vi "SEN_Loop.vi"() -> ()   [LabVIEW 2020, in "PigeonIMU_SEN_ts.lvlib"]
uses:
  PigeonIMU_SEN_ts.lvlib
  <vilib>/Rock Robotics/WPI/ThirdParty/Phoenix-LabVIEW/Pigeon2/controls/CTRE_Phoenix_Pigeon2_Configurables.ctl
  Cluster_CMD_SEN_Data.ctl
  Shared Code/TypeDefs/Cluster_Unity Yaw-Pitch-Roll.ctl
  Shared Code/TypeDefs/Dial_Compase heading unit circle CCW positive.ctl
  ENUM_SEN_State.ctl
  <vilib>/Rock Robotics/WPI/ThirdParty/Phoenix-LabVIEW/Pigeon IMU/CTRE_PigeonIMU_DeviceRef.ctl
  <vilib>/Rock Robotics/WPI/ThirdParty/Phoenix-LabVIEW/Pigeon IMU/CTRE_PigeonIMU_ConnectionType.ctl
  ENUM_SEN_Action.ctl
  ca1e8ace-5cb3-4d4b-8a00-bfa7a3df30b2.vi
  Global_CMD_SEN_Data In.vi
  RoboRIO Utilities/Global_STOP.vi
  Global_SEN_Data Out.vi
  <vilib>/Rock Robotics/WPI/ThirdParty/Phoenix-LabVIEW/Pigeon2/CTRE_Phoenix_Pigeon2_GetGravityVector.vi
  <vilib>/Rock Robotics/WPI/ThirdParty/Phoenix-LabVIEW/Pigeon IMU/CTRE_PigeonIMU_GetRawGyro.vi
  <vilib>/Rock Robotics/WPI/ThirdParty/Phoenix-LabVIEW/Pigeon IMU/CTRE_PigeonIMU_GetFusedHeading.vi
  <vilib>/Rock Robotics/WPI/ThirdParty/Phoenix-LabVIEW/Pigeon IMU/CTRE_PigeonIMU_GetBiasedAccelerometer.vi
panel:
  out "Pigeon Running":bool
  out "YawPitchRoll":T1 {"Roll" scale format="%.3f"; "Pitch" scale format="%.3f"; "Yaw" scale format="%.3f"}
  in  "CMD_SEN_Pigeon_Data":T3
  in  "Set Values":bool
  in  "Pigeon2 Config":T4
  out "Pigeon Ready":bool
  out "Pigeon Enabled":bool
  out "Cycle Time (S)":dbl format="%.3g"
  # "Yaw Angle needed to reach the current orientation in degrees"
  # "Configures the mounting pose of the Pigeon2\nThis is the yaw-pitch-roll teh Pigeon2 underwent to get to its current orientation,\n referenced from the robot's point of view\nThis is only necessary if the Pigeon2 is mounted at an exotic angle near the gimbal lock point or not forward.\nIf the pigeon is relatively flat and pointed forward, this is not needed"
  # "Pitch Angle needed to reach the current orientation in degrees"
  # "Roll Angle needed to reach the current orientation in degrees"
  # "Disables the temperature compensation\nfrom the Pigeon2. It is recommended that\nthis remains false"
  # "Disables the no-motion calibration from the\nPigeon2. It is recommended that this \nremains false"
  # "Enables the compass for Pigeon2\nThis is not recommended for any indoor robotics"
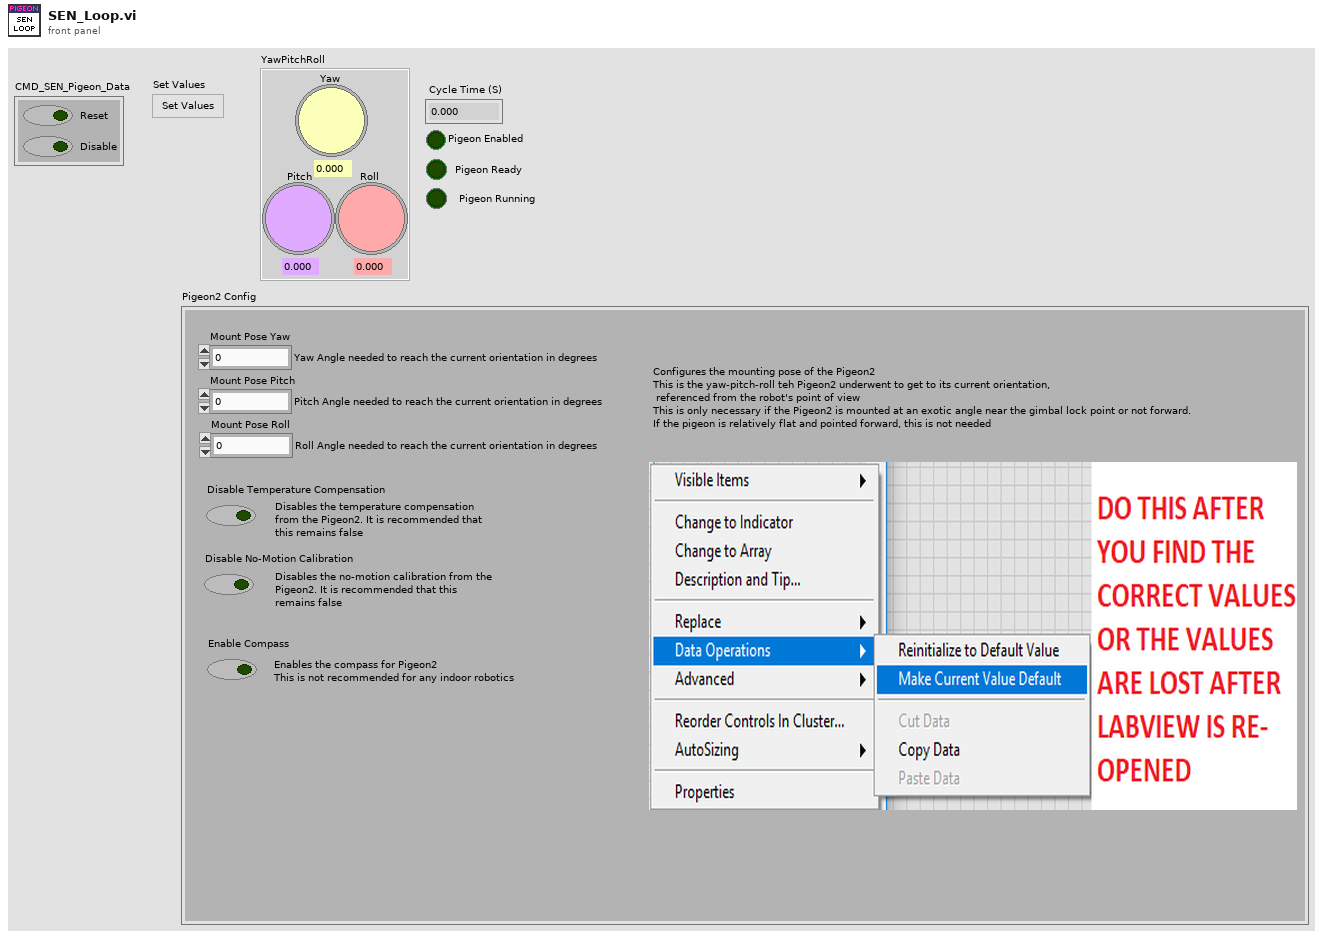
[diagram p1: front panel]
types:
  T1 = typedef "Cluster_Unity Yaw-Pitch-Roll.ctl" = cluster{"Yaw":T2, "Pitch":T2, "Roll":T2}
  T2 = typedef "Dial_Compase heading unit circle CCW positive.ctl" = dbl
  T3 = typedef "PigeonIMU_SEN_ts.lvlib/Cluster_CMD_SEN_Data.ctl" = cluster{"Reset":bool, "Disable":bool}
  T4 = typedef "CTRE_Phoenix_Pigeon2_Configurables.ctl" = cluster{"Mount Pose Yaw":dbl, "Mount Pose Pitch":dbl, "Mount Pose Roll":dbl, "Disable Temperature Compensation":bool, "Disable No-Motion Calibration":bool, "Enable Compass":bool}
  T5 = cluster{"Heading":dbl, "Valid?":bool, "Fusing?":bool}
  T6 = typedef "CTRE_PigeonIMU_DeviceRef.ctl" = cluster{"DeviceStatus":errorcluster, "Device Number":u8, "Type":T7, "Device ID":u32, "Handle":u64, "UsageFrame":u32, "Library Path":path}
  T7 = typedef "CTRE_PigeonIMU_ConnectionType.ctl" = u32
  T8 = typedef "PigeonIMU_SEN_ts.lvlib/ENUM_SEN_State.ctl" = enum16{"Starting", "Reseting", "Enableing", "Disabeling", "Shutting Down"}
  T9 = cluster{"PigeonIMUDevRef":T6, "State":T8, "Previous State":T8, "Current Time":timestamp, "Previous Time":timestamp, "Start Time":timestamp, "Target Time (ms)":u32, "Cycle Time(S)":dbl, "Reset":bool, "Yaw Pitch Roll":T1, "Fused Heading":cluster{"Heading":dbl, "Valid?":bool, "Fusing?":bool}, "IMU Ready":bool, "Swing Threshold":dbl, "Swinging":bool, "Swing Array Size":i32, "CMD_SEN_Pigeon_Data":T3}
  T10 = typedef "PigeonIMU_SEN_ts.lvlib/ENUM_SEN_Action.ctl" = enum16{"No Action", "Reset Time", "Zero Heading", "Read Heading", "Read Raw ", "Configure IMU", "Check IMU Reset", "Set Enable Cycle Time", "Set Disable Cycle Time"}
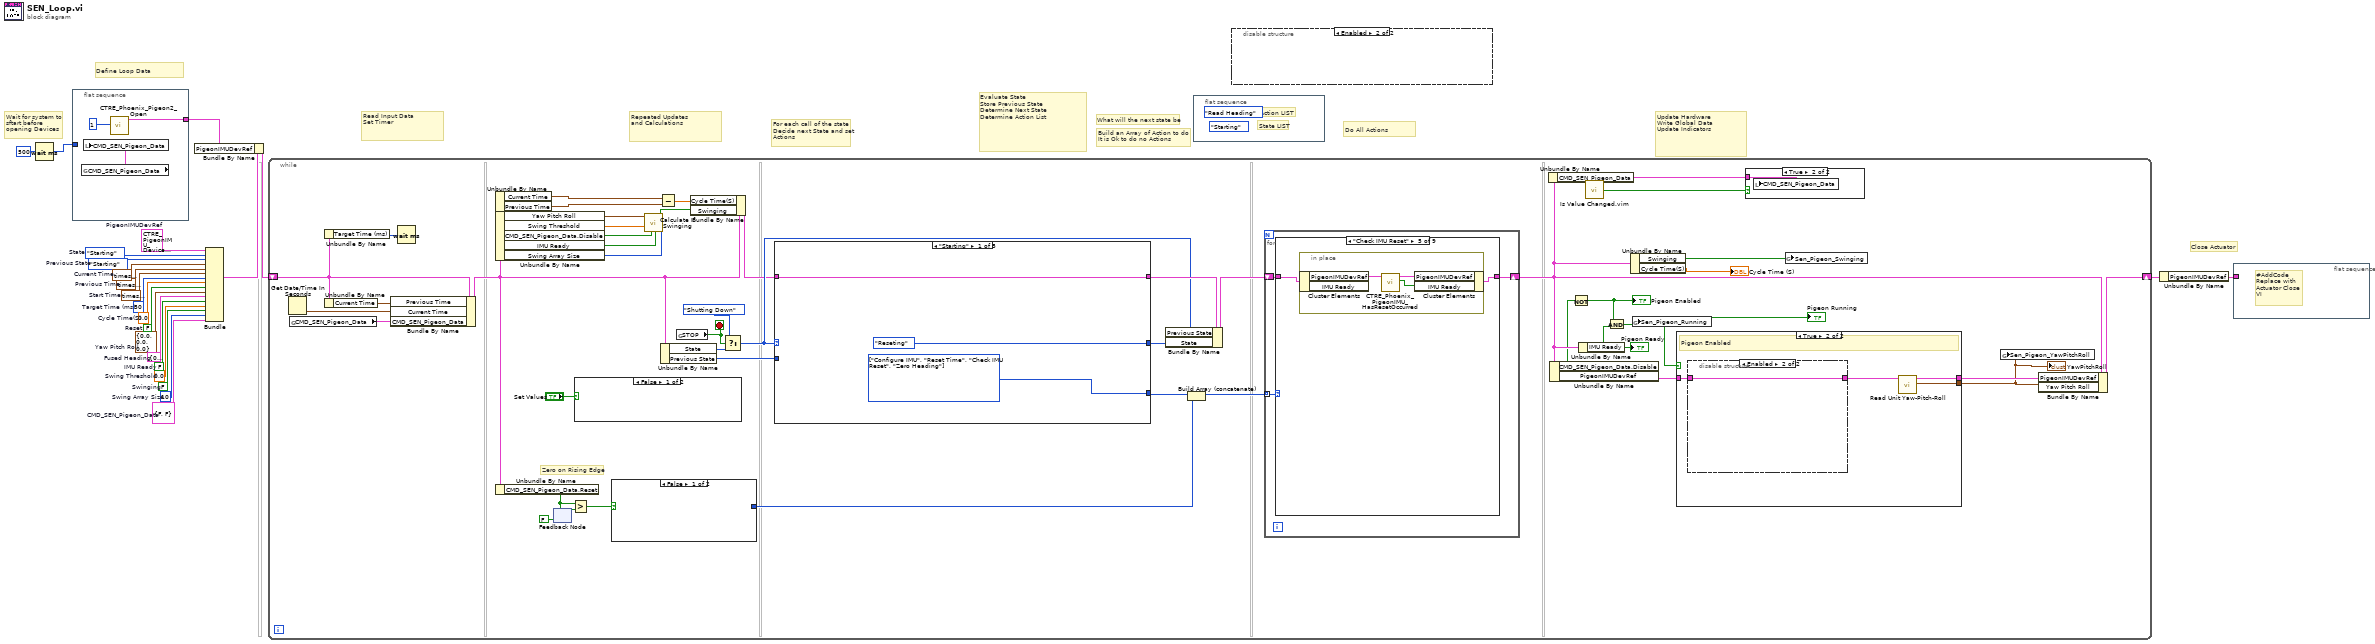
[diagram p0: block diagram]
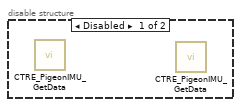
[diagram p2: hidden frame]
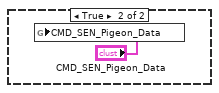
[diagram p4: hidden frame]
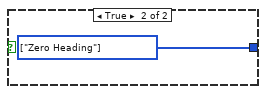
[diagram p5: hidden frame]
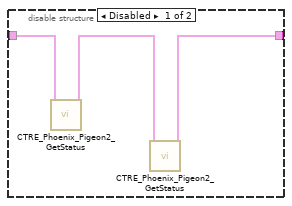
[diagram p7: hidden frame]
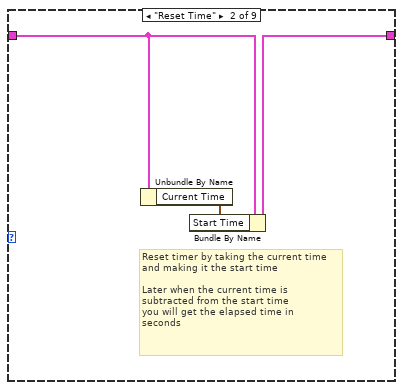
[diagram p9: hidden frame]
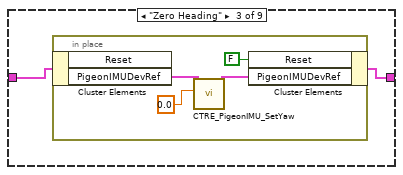
[diagram p10: hidden frame]
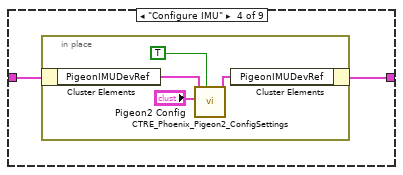
[diagram p11: hidden frame]
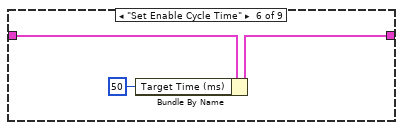
[diagram p12: hidden frame]
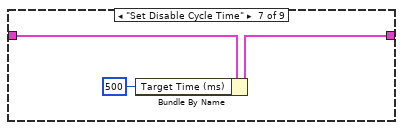
[diagram p13: hidden frame]
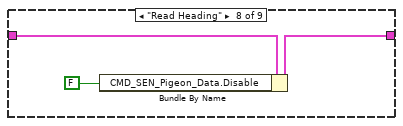
[diagram p14: hidden frame]
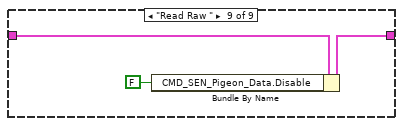
[diagram p15: hidden frame]
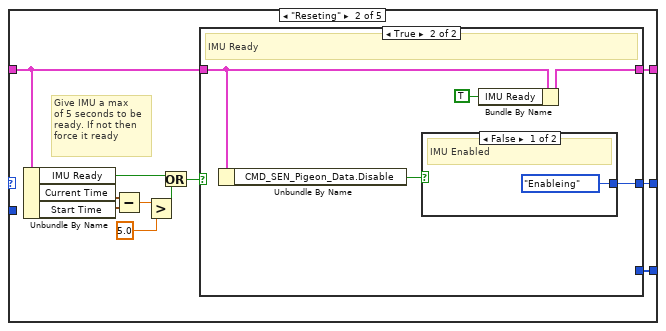
[diagram p16: hidden frame]
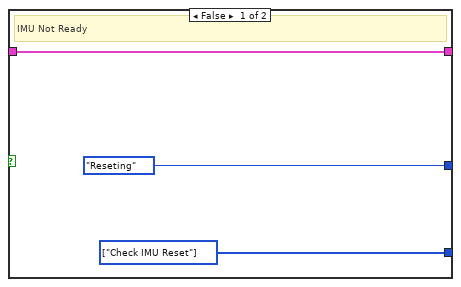
[diagram p17: hidden frame]
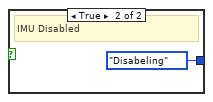
[diagram p18: hidden frame]
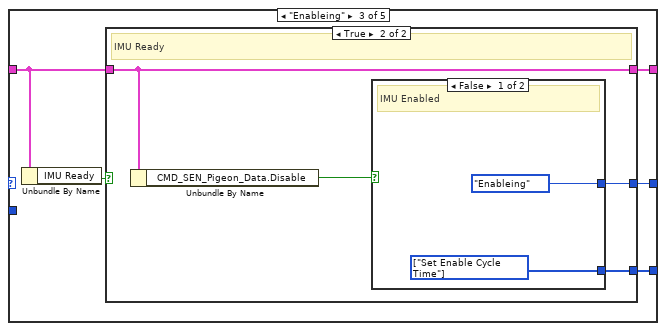
[diagram p19: hidden frame]
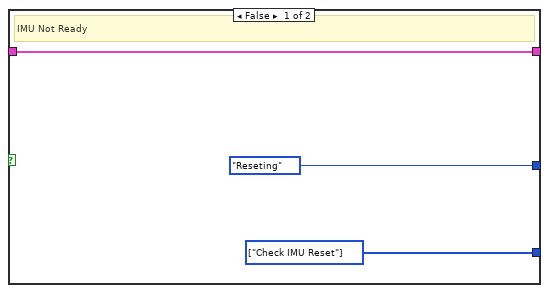
[diagram p20: hidden frame]
diagram:
  w1 = T1 {"Yaw"=0.0, "Pitch"=0.0, "Roll"=0.0}  # Yaw Pitch Roll
  w2 = T3 {"Reset"=FALSE, "Disable"=FALSE}  # CMD_SEN_Pigeon_Data
  w3 = 10  # Swing Array Size
  w4 = FALSE  # Swinging
  w5 = 0.0  # Swing Threshold
  w6 = FALSE  # IMU Ready
  w7 = T5 {"Heading"=0.0, "Valid?"=FALSE, "Fusing?"=FALSE}  # Fused Heading
  w8 = T6 {"DeviceStatus"={"status"=FALSE, "code"=0, "source"=""}, "Device Number"=0, "Type"=352321536, "Device ID"=0, "Handle"=0, "UsageFrame"=0, "Library Path"=path ""}  # PigeonIMUDevRef
  w16 = 0.0  # Cycle Time(S)
  w17 = ENUM_SEN_State."Starting"  # Previous State
  w18 = timestamp(0 s since 1904-01-01)  # Previous Time
  w19 = u32 50  # Target Time (ms)
  w20 = FALSE  # Reset
  w21 = timestamp(0 s since 1904-01-01)  # Start Time
  w22 = timestamp(0 s since 1904-01-01)  # Current Time
  w23 = ENUM_SEN_State."Starting"  # State
  # "Wait for system to\nsftart before\nopening Devices"
  # "Build an Array of Action to do\nIt is Ok to do no Actions"
  # "What will the next state be"
  # "For each call of the state\nDecide next State and set\nActions"
  # "Close Actuator"
  # "Define Loop Data"
  # "Repeated Updates\nand Calculations"
  # "Read Input Data\nSet Timer"
  # "Evaluate State\nStore Previous State\nDetermine Next State\nDetermine Action List"
  # "Do All Actions"
  # "Update Hardware\nWrite Global Data\nUpdate Indicators"
  n1 = Wait (ms)(milliseconds to wait=u32 500) -> (millisecond timer value=w9:u32)
  n2 = flat-sequence {
    tunnel: [w26] -> w11
    tunnel: w9 -> [_]
    frame #0 {
      n3 = global read "Global_CMD_SEN_Data In.vi" "CMD_SEN_Pigeon_Data"() -> (w24:T3)
      n4 = local write "CMD_SEN_Pigeon_Data"(w24) -> ()
      n5 = call <vilib>:"CTRE_Phoenix_Pigeon2_Open.vi"("Device Number"=u8 1) -> ("PigeonIMUDevRef"=w26:T6)  [unwired: 9 in, 1 out]
    }
  }
  n6 = Bundle("PigeonIMUDevRef"=w8, "State"=w23, "Previous State"=w17, "Current Time"=w22, "Previous Time"=w18, "Start Time"=w21, "Target Time (ms)"=w19, "Cycle Time(S)"=w16, "Reset"=w20, "Yaw Pitch Roll"=w1, "Fused Heading"=w7, "IMU Ready"=w6, "Swing Threshold"=w5, "Swinging"=w4, "Swing Array Size"=w3, "CMD_SEN_Pigeon_Data"=w2) -> (w13:T9)  [unwired: 1 in]
  n7 = Bundle By Name(cluster=w13, "PigeonIMUDevRef"=w11) -> (w12:T9)
  n8 = while {
    shift-right: [w54] -> w14
    shift-left: w12 -> [w52]
    stop <- w67 stop-if-true
    # "Zero on Rising Edge"
    n9 = Get Date/Time In Seconds() -> (seconds since 1Jan1904=w71:timestamp)
    n10 = global read "Global_CMD_SEN_Data In.vi" "CMD_SEN_Pigeon_Data"() -> (w31:T3)
    n11 = Unbundle By Name(w52) -> ("Target Time (ms)"=w64:u32)
    n12 = Unbundle By Name(w52) -> ("Current Time"=w63:timestamp)
    n13 = Bundle By Name(cluster=w52, "Previous Time"=w63, "Current Time"=w71, "CMD_SEN_Pigeon_Data"=w31) -> (w43:T9)
    n14 = Wait (ms)(milliseconds to wait=w64) -> ()  [unwired: 1 out]
    n15 = Unbundle By Name(w43) -> ("Current Time"=w45:timestamp, "Previous Time"=w60:timestamp)
    n16 = Unbundle By Name(w43) -> ("Yaw Pitch Roll"=w38:T1, "Swing Threshold"=w41:dbl, "CMD_SEN_Pigeon_Data.Disable"=w39:bool, "IMU Ready"=w40:bool, "Swing Array Size"=w37:i32)
    n17 = Unbundle By Name(w43) -> ("CMD_SEN_Pigeon_Data.Reset"=w49:bool)
    n18 = feedback-in #1(w49) -> ()
    n19 = feedback #1(FALSE ("CMD_SEN_Pigeon_Reset")) -> (w50:bool)
    n20 = Greater?(x=w49, y=w50) -> (0:w48:bool)
    n21 = case shown="False" "Set Values" {
      frame False {
      }
      frame True {
        n22 = global write "Global_CMD_SEN_Data In.vi" "CMD_SEN_Pigeon_Data"("CMD_SEN_Pigeon_Data") -> ()
      }
    }
    n23 = case shown="False" w48 {
      tunnel: [_ w74] -> w46
      frame False {
      }
      frame True {
        w74 = T10[] [enum."Zero Heading"] items=["No Action", "Reset Time", "Zero Heading", "Read Heading", "Read Raw ", "Configure IMU", "Check IMU Reset", "Set Enable Cycle Time", "Set Disable Cycle Time"] ("Actions")
      }
    }
    n24 = call "Calculate If Swinging.vi"("Swing Array Size"=w37, "IMU Ready"=w40, "Disable"=w39, "Swing Threshold"=w41, "Yaw Pich Roll"=w38) -> ("Swinging Out"=w42:bool)  [unwired: 6 in]
    n25 = Subtract(x=w45, y=w60) -> (x-y=w58:dbl)
    n26 = Unbundle By Name(w43) -> ("State"=w65:T8, "Previous State"=w62:T8)
    n27 = global read "Global_STOP.vi" "STOP"() -> (w67:bool)
    n28 = Bundle By Name(cluster=w43, "Cycle Time(S)"=w58, "Swinging"=w42) -> (w59:T9)
    n29 = Select(t=ENUM_SEN_State."Shutting Down" ("State"), s=w67, f=w65) -> (s? t:f=w61:T8)
    n30 = case shown="\"Starting\"" w61 {
      tunnel: w59 -> [w122 w132 w147 w162 w175]
      tunnel: [w122 w131 w146 w161 w175] -> w69
      tunnel: [ENUM_SEN_State."Reseting" ("State") w130 w145 w160 ENUM_SEN_State."Shutting Down" ("State")] -> w68
      tunnel: [w120 w129 w144 w159 _] -> w57
      tunnel: w62 -> [_ _ _ _ _]
      frame "Starting" {
        w120 = T10[] [enum."Configure IMU", enum."Reset Time", enum."Check IMU Reset", enum."Zero Heading"] items=["No Action", "Reset Time", "Zero Heading", "Read Heading", "Read Raw ", "Configure IMU", "Check IMU Reset", "Set Enable Cycle Time", "Set Disable Cycle Time"] ("Actions")
      }
      frame "Reseting" {
        # "Give IMU a max\nof 5 seconds to be\nready. If not then\nforce it ready"
        n31 = Unbundle By Name(w132) -> ("IMU Ready"=w133:bool, "Current Time"=w128:timestamp, "Start Time"=w127:timestamp)
        n32 = Subtract(x=w128, y=w127) -> (x-y=w126:dbl)
        n33 = Greater?(x=w126, y=5.0) -> (0:w123:bool)
        n34 = Or(x=w133, y=w123) -> (x .or. y?=w124:bool)
        n35 = case shown="True" w124 {
          tunnel: w132 -> [w134 w138]
          tunnel: [w134 w139] -> w131
          tunnel: [ENUM_SEN_State."Reseting" ("State") w141] -> w130
          tunnel: [w135 _] -> w129
          frame False {
            w135 = T10[] [enum."Check IMU Reset"] items=["No Action", "Reset Time", "Zero Heading", "Read Heading", "Read Raw ", "Configure IMU", "Check IMU Reset", "Set Enable Cycle Time", "Set Disable Cycle Time"] ("Actions")
            # "IMU Not Ready"
          }
          frame True {
            # "IMU Ready"
            n36 = Unbundle By Name(w138) -> ("CMD_SEN_Pigeon_Data.Disable"=w140:bool)
            n37 = case shown="False" w140 {
              tunnel: [ENUM_SEN_State."Enableing" ("State") ENUM_SEN_State."Disabeling" ("State")] -> w141
              frame False {
                # "IMU Enabled"
              }
              frame True {
                # "IMU Disabled"
              }
            }
            n38 = Bundle By Name(cluster=w138, "IMU Ready"=TRUE) -> (w139:T9)
          }
        }
      }
      frame "Enableing" {
        n39 = Unbundle By Name(w147) -> ("IMU Ready"=w148:bool)
        n40 = case shown="True" w148 {
          tunnel: w147 -> [w149 w154]
          tunnel: [w149 w154] -> w146
          tunnel: [ENUM_SEN_State."Reseting" ("State") w155] -> w145
          tunnel: [w150 w152] -> w144
          frame False {
            w150 = T10[] [enum."Check IMU Reset"] items=["No Action", "Reset Time", "Zero Heading", "Read Heading", "Read Raw ", "Configure IMU", "Check IMU Reset", "Set Enable Cycle Time", "Set Disable Cycle Time"] ("Actions")
            # "IMU Not Ready"
          }
          frame True {
            # "IMU Ready"
            n41 = Unbundle By Name(w154) -> ("CMD_SEN_Pigeon_Data.Disable"=w153:bool)
            n42 = case shown="False" w153 {
              tunnel: [ENUM_SEN_State."Enableing" ("State") ENUM_SEN_State."Disabeling" ("State")] -> w155
              tunnel: [w156 _] -> w152
              frame False {
                w156 = T10[] [enum."Set Enable Cycle Time"] items=["No Action", "Reset Time", "Zero Heading", "Read Heading", "Read Raw ", "Configure IMU", "Check IMU Reset", "Set Enable Cycle Time", "Set Disable Cycle Time"] ("Actions")
                # "IMU Enabled"
              }
              frame True {
                # "IMU Disabled"
              }
            }
          }
        }
      }
      frame "Disabeling" {
        n43 = Unbundle By Name(w162) -> ("IMU Ready"=w163:bool)
        n44 = case shown="True" w163 {
          tunnel: w162 -> [w164 w169]
          tunnel: [w164 w169] -> w161
          tunnel: [ENUM_SEN_State."Reseting" ("State") w170] -> w160
          tunnel: [w165 w167] -> w159
          frame False {
            w165 = T10[] [enum."Check IMU Reset"] items=["No Action", "Reset Time", "Zero Heading", "Read Heading", "Read Raw ", "Configure IMU", "Check IMU Reset", "Set Enable Cycle Time", "Set Disable Cycle Time"] ("Actions")
            # "IMU Not Ready"
          }
          frame True {
            # "IMU Ready"
            n45 = Unbundle By Name(w169) -> ("CMD_SEN_Pigeon_Data.Disable"=w168:bool)
            n46 = case shown="True" w168 {
              tunnel: [ENUM_SEN_State."Enableing" ("State") ENUM_SEN_State."Disabeling" ("State")] -> w170
              tunnel: [_ w172] -> w167
              frame False {
                # "IMU Enabled"
              }
              frame True {
                w172 = T10[] [enum."Set Disable Cycle Time"] items=["No Action", "Reset Time", "Zero Heading", "Read Heading", "Read Raw ", "Configure IMU", "Check IMU Reset", "Set Enable Cycle Time", "Set Disable Cycle Time"] ("Actions")
                # "IMU Disabled"
              }
            }
          }
        }
      }
      frame "Shutting Down" {
      }
    }
    n47 = Bundle By Name(cluster=w69, "Previous State"=w61, "State"=w68) -> (w70:T9)
    n48 = Build Array (concatenate)(w57, w46) -> (w47:T10[])
    n49 = for {
      tunnel: w47 -> [w86] mode=indexing
      shift-right: [w85] -> w33
      shift-left: w70 -> [w84]
      n50 = case shown="\"Check IMU Reset\"" w86 {
        tunnel: w84 -> [w87 w90 w92 w98 w104 w109 w112 w116 w119]
        tunnel: [w87 w89 w91 w97 w103 w110 w113 w115 w118] -> w85
        frame "No Action" {
        }
        frame "Reset Time" {
          # "Reset timer by taking the current time\nand making it the start time\n\nLater when the current time is \nsubtracted from the start time\nyou will get the elapsed time in \nseconds"
          n51 = Unbundle By Name(w90) -> ("Current Time"=w88:timestamp)
          n52 = Bundle By Name(cluster=w90, "Start Time"=w88) -> (w89:T9)
        }
        frame "Zero Heading" {
          n53 = in-place {
            n54 = in-place-cluster #2(w92) -> ("PigeonIMUDevRef"=w95:T6)  [unwired: 1 out]
            n55 = call <vilib>:"CTRE_PigeonIMU_SetYaw.vi"("Value"=0.0, "PigeonIMUDevRef"=w95) -> ("PigeonIMUDevRef"=w94:T6)  [unwired: 8 in, 1 out]
            n56 = in-place-cluster #2("Reset"=FALSE, "PigeonIMUDevRef"=w94) -> (w91:T9)
          }
        }
        frame "Configure IMU" {
          n57 = in-place {
            n58 = in-place-cluster #3(w98) -> ("PigeonIMUDevRef"=w102:T6)
            n59 = call <vilib>:"CTRE_Phoenix_Pigeon2_ConfigSettings.vi"("Force Write"=TRUE, "Pigeon2 Configurables"="Pigeon2 Config", "PigeonIMUDevRef 2"=w102) -> ("PigeonIMUDevRef"=w101:T6)  [unwired: 7 in, 1 out]
            n60 = in-place-cluster #3("PigeonIMUDevRef"=w101) -> (w97:T9)
          }
        }
        frame "Check IMU Reset" {
          n61 = in-place {
            n62 = in-place-cluster #4(w104) -> ("PigeonIMUDevRef"=w107:T6)  [unwired: 1 out]
            n63 = call <vilib>:"CTRE_Phoenix_PigeonIMU_HasResetOccurred.vi"("CTRE_PigeonIMU_DeviceRef"=w107) -> ("Has Reset Occurred?"=w105:bool, "CTRE_PigeonIMU_DeviceRef"=w106:T6)  [unwired: 8 in, 1 out]
            n64 = in-place-cluster #4("PigeonIMUDevRef"=w106, "IMU Ready"=w105) -> (w103:T9)
          }
        }
        frame "Set Enable Cycle Time" {
          n65 = Bundle By Name(cluster=w109, "Target Time (ms)"=u32 50) -> (w110:T9)
        }
        frame "Set Disable Cycle Time" {
          n66 = Bundle By Name(cluster=w112, "Target Time (ms)"=u32 500) -> (w113:T9)
        }
        frame "Read Heading" {
          n67 = Bundle By Name(cluster=w116, "CMD_SEN_Pigeon_Data.Disable"=FALSE ("Read Enable")) -> (w115:T9)
        }
        frame "Read Raw " {
          n68 = Bundle By Name(cluster=w119, "CMD_SEN_Pigeon_Data.Disable"=FALSE ("Read Enable")) -> (w118:T9)
        }
      }
    }
    n69 = Unbundle By Name(w33) -> ("CMD_SEN_Pigeon_Data"=w34:T3)
    n70 = Unbundle By Name(w33) -> ("CMD_SEN_Pigeon_Data.Disable"=w30:bool, "PigeonIMUDevRef"=w56:T6)
    n71 = Not(x=w30) -> (.not. x?=w29:bool)
    "Pigeon Enabled" <- w29
    n72 = Unbundle By Name(w33) -> ("IMU Ready"=w44:bool)
    "Pigeon Ready" <- w44
    n73 = call "Is Value Changed.vim"("value"=w34) -> ("changed or first call?"=w35:bool)
    n74 = And(x=w29, y=w44) -> (x .and. y?=w28:bool)
    "Pigeon Running" <- w28
    n75 = Unbundle By Name(w33) -> ("Swinging"=w36:bool, "Cycle Time(S)"=→"Cycle Time (S)":dbl)
    n76 = global write "Global_SEN_Data Out.vi" "Sen_Pigeon_Running"(w28) -> ()
    n77 = case shown="True" w28 {
      tunnel: w56 -> [w75 w76]
      tunnel: [w75 w79] -> w55
      tunnel: [_ w78] -> w27
      frame False {
        # "Pigeon Disabled"
      }
      frame True {
        # "Pigeon Enabled"
        n78 = disable-structure shown="Enabled" {
          disable-tunnel: [w80 w83] -> w77
          disable-tunnel: w76 -> [w82 w83]
          frame Disabled {
            n79 = call-poly <vilib>:"CTRE_Phoenix_Pigeon2_GetStatus.vi"("PigeonIMUDevRef 2"=w82) -> ("PigeonIMUDevRef"=w81:T6)  [unwired: 8 in, 2 out]
            n80 = call-poly <vilib>:"CTRE_Phoenix_Pigeon2_GetStatus.vi"("PigeonIMUDevRef"=w81) -> ("PigeonIMUDevRef"=w80:T6)  [unwired: 8 in, 2 out]
          }
          frame Enabled {
          }
        }
        n81 = call "Read Unit Yaw-Pitch-Roll.vi"("PigeonIMUDevRef"=w77) -> ("Unit Yaw-Pitch-Roll Out"=w78:T1, "PigeonIMUDevRef Out"=w79:T6)  [unwired: 8 in, 1 out]
      }
    }
    "YawPitchRoll" <- w27
    n82 = case shown="True" w35 {
      tunnel: w34 -> [_ w72]
      frame False {
      }
      frame True {
        n83 = local write "CMD_SEN_Pigeon_Data"(w72) -> ()
      }
    }
    n84 = global write "Global_SEN_Data Out.vi" "Sen_Pigeon_Swinging"(w36) -> ()
    n85 = global write "Global_SEN_Data Out.vi" "Sen_Pigeon_YawPitchRoll"(w27) -> ()
    n86 = Bundle By Name(cluster=w33, "PigeonIMUDevRef"=w55, "Yaw Pitch Roll"=w27) -> (w54:T9)
  }
  n87 = flat-sequence {
    frame #0 {
      (unwired) ENUM_SEN_State."Starting" ("State")
      (unwired) ENUM_SEN_Action."Read Heading" ("Action")
      # "State LIST"
      # "Action LIST"
    }
  }
  n88 = disable-structure shown="Enabled" {
    frame Disabled {
      n89 = call-poly <vilib>:"CTRE_PigeonIMU_GetData.vi"() -> ()  [unwired: 9 in, 3 out]
      n90 = call-poly <vilib>:"CTRE_PigeonIMU_GetData.vi"() -> ()  [unwired: 9 in, 3 out]
    }
    frame Enabled {
    }
  }
  n91 = Unbundle By Name(w14) -> ("PigeonIMUDevRef"=w15:T6)
  n92 = flat-sequence {
    tunnel: w15 -> [_]
    frame #0 {
      # "#AddCode\nReplace with \nActuator Close\nVI"
    }
  }
